vi "MST_softwareBin.vi"() -> ()   [LabVIEW 2012]
uses:
  <vilib>/addons/database/Auxilliary.llb/DB Tools Cursor Type.ctl
  <vilib>/Utility/NIReport.llb/NI_report.lvclass
  <vilib>/addons/database/Connection.llb/DB Tools Open Connec (Path).vi
  <vilib>/addons/database/Connection.llb/Conn Execute.vi
  <vilib>/addons/database/Recordset.llb/Rec Fetch Recordset Data (R).vi
  <vilib>/addons/database/Recordset.llb/Rec Destroy - Connection.vi
  <vilib>/Utility/NIReport.llb/Append Text Table to Report (wrap).vi
  <vilib>/addons/database/_DB Variant To Data/Database Variant To Data.xnode
  <vilib>/addons/database/NI_Database_API.lvlib
  <vilib>/Utility/NIReport.llb/Excel/NI_Excel.lvclass
panel:
  out "error out 2":errorcluster
  out "Row Headers":string[](array[string])
  in  "Report Template":path=path "O:/Monitor/Report/MSTsoftBin.xls"
  out "appended array":string[](array[string])
  out "data":string
  out "recordset data":variant[][](array[variant])
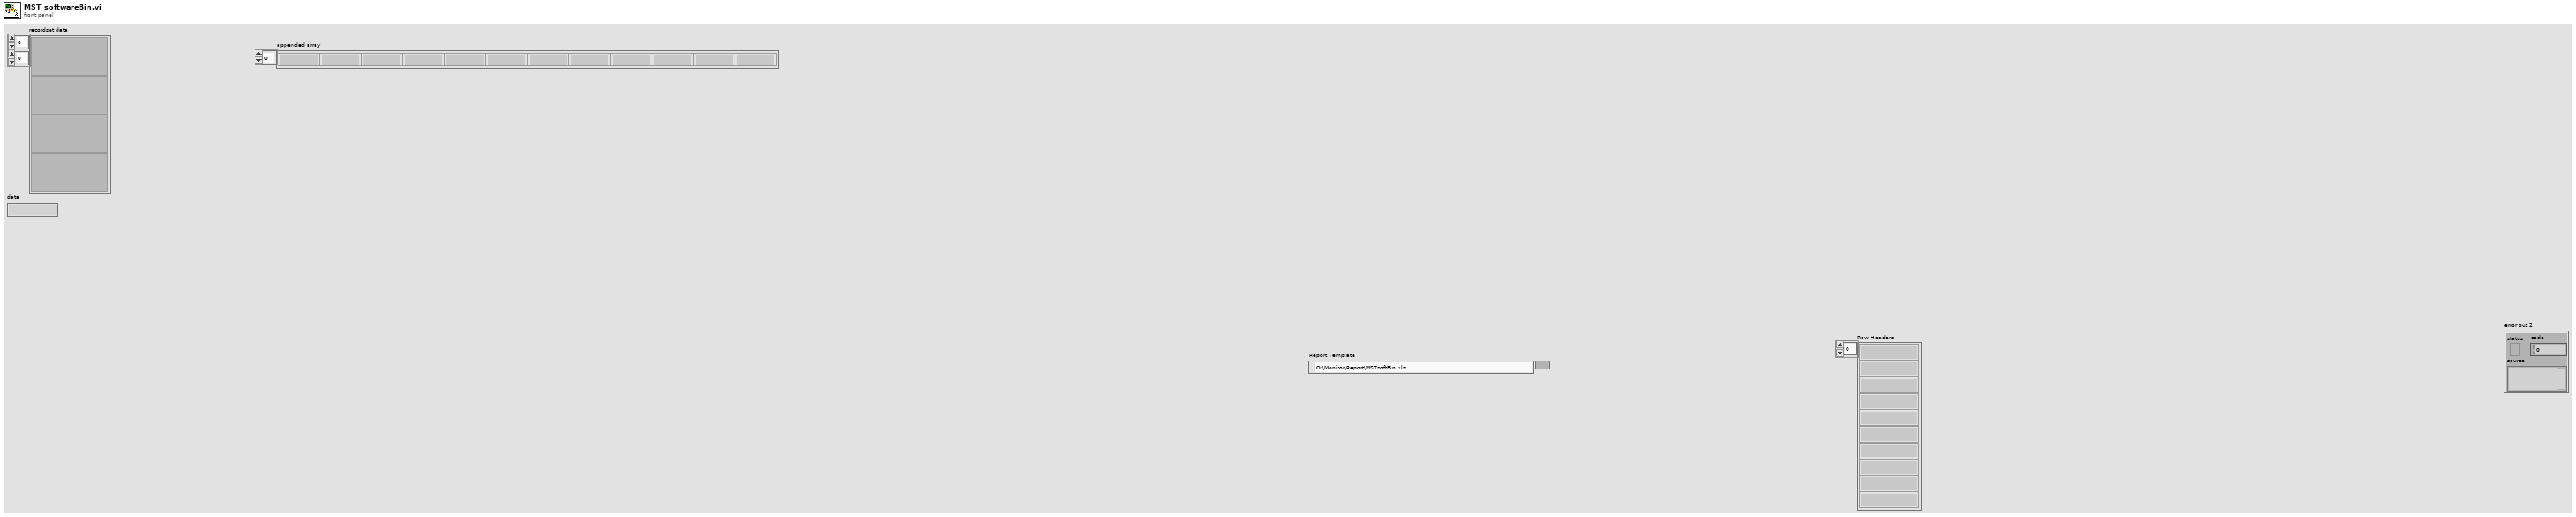
[diagram p1: front panel]
types:
  T1 = typedef "NI_Database_API.lvlib/DB Tools Cursor Type.ctl" = enum16{"forward-only", "keyset", "dynamic", "static"}
  T2 = enum16{"Standard Report", "HTML", "Word", "Excel"}
  T3 = typedef "NI_Database_API.lvlib/Conn ObjectReference.ctl" = refnum<k1>
  T4 = typedef "NI_Database_API.lvlib/Rec ObjectReference.ctl" = refnum<k1>
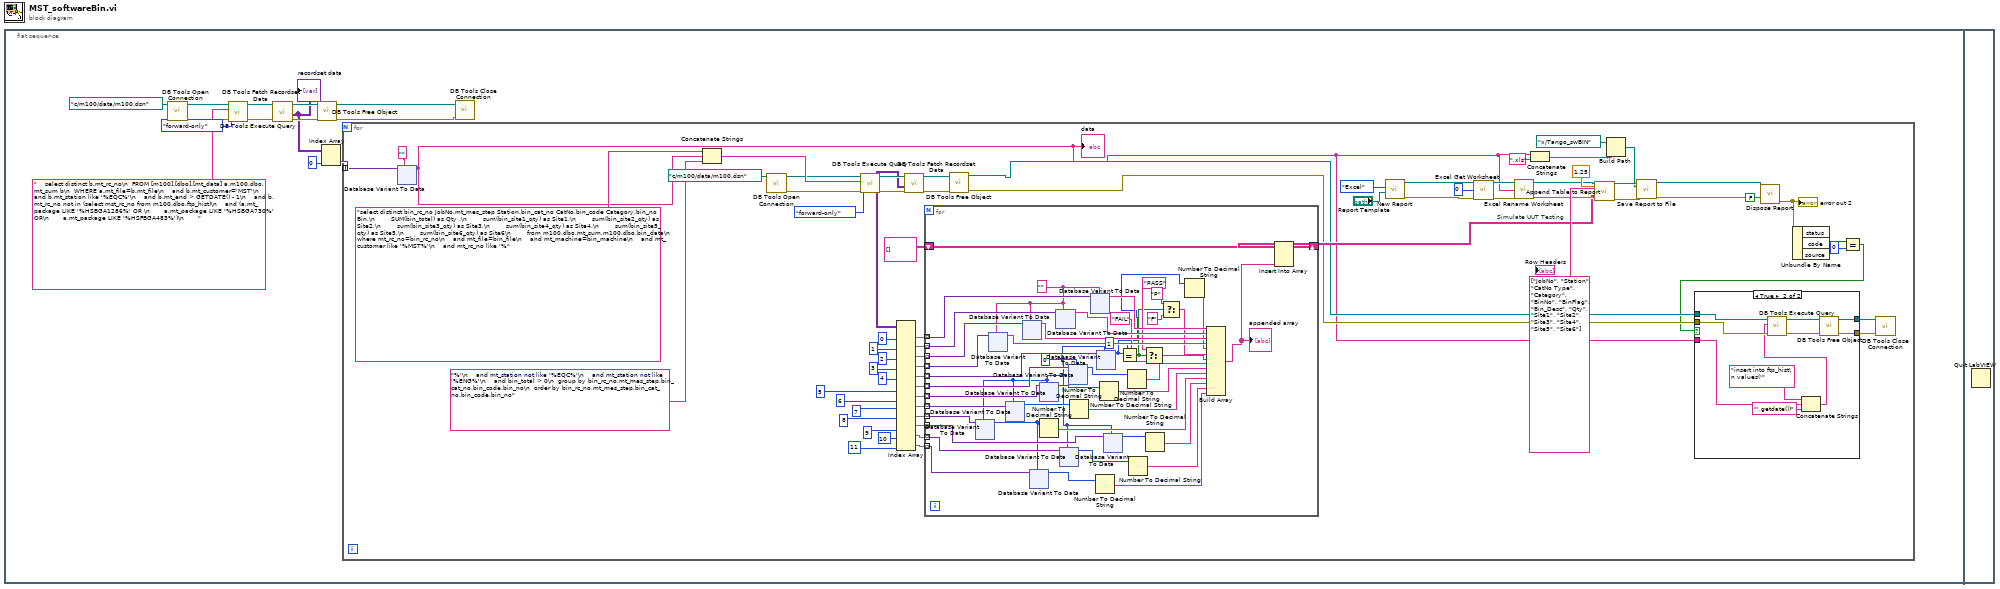
[diagram p0: block diagram]
diagram:
  n1 = flat-sequence {
    frame #0 {
      n2 = call-poly <vilib>:"DB Tools Open Connection.vi"("connection information"=path "c:/m100/data/m100.dsn") -> ("error out"=w11:errorcluster, "connection reference"=w14:T3)  [unwired: 7 in]
      n3 = call-poly <vilib>:"DB Tools Execute Query.vi"("error in (no error)"=w11, "cursor type"=DB_Tools_Cursor_Type."forward-only", "SQL query"="    select distinct b.mt_rc_no\n  FROM [m100].[dbo].[mt_data] a,m100.dbo.mt_sum b\n  WHERE a.mt_file=b.mt_file\n    and b.mt_customer='MST'\n    and b.mt_station like '%EQC%'\n    and b.mt_end > GETDATE() - 1\n    and b.mt_rc_no not in (select mst_rc_no from m100.dbo.ftp_hist)\n    and (a.mt_package LIKE '%HSBGA1286%' OR \n       a.mt_package LIKE '%HSBGA730%' OR\n       a.mt_package LIKE '%HSFBGA483%')\n       ", "connection reference"=w14) -> ("error out"=w10:errorcluster, "recordset reference"=w13:T4)  [unwired: 4 in]
      n4 = call-poly <vilib>:"DB Tools Fetch Recordset Data.vi"("error in (no error)"=w10, "recordset reference"=w13) -> ("error out"=w9:errorcluster, "recordset data"=w5:variant[][], "recordset reference out"=w12:T4)  [unwired: 3 in]
      "recordset data" <- w5
      n5 = call-poly <vilib>:"DB Tools Free Object.vi"("error in (no error)"=w9, "recordset reference"=w12) -> ("error out"=w1:errorcluster, "connection reference"=w2:T3)  [unwired: 8 in]
      n6 = Index Array(array=w5, index (col)=0 ("disabled index (col)")) -> (element=w3:variant[])  [unwired: 1 in]
      n7 = for {
        tunnel: w3 -> [w83] mode=indexing
        # "Simulate UUT Testing"
        n8 = xnode "Database Variant To Data"("database variant"=w83, "type"="") -> ("data"=w23:string)  [unwired: 1 in, 1 out]
        "data" <- w23
        n9 = Concatenate Strings("select distinct bin_rc_no JobNo,mt_mes_step Station,bin_cat_no CatNo,bin_code Category,bin_no Bin,\n        SUM(bin_total) as Qty ,\n        sum(bin_site1_qty) as Site1,\n        sum(bin_site2_qty) as Site2,\n        sum(bin_site3_qty) as Site3,\n        sum(bin_site4_qty) as Site4,\n        sum(bin_site5_qty) as Site5,\n        sum(bin_site6_qty) as Site6\n        from m100.dbo.mt_sum,m100.dbo.bin_data\n  where mt_rc_no=bin_rc_no\n    and mt_file=bin_file\n    and mt_machine=bin_machine\n    and mt_customer like '%MST%'\n    and mt_rc_no like '%" ("string"), w23, "%'\n    and mt_station not like '%EQC%'\n    and mt_station not like '%ENG%'\n    and bin_total > 0\n  group by bin_rc_no,mt_mes_step,bin_cat_no,bin_code,bin_no\n  order by bin_rc_no,mt_mes_step,bin_cat_no,bin_code,bin_no" ("string")) -> (w74:string)
        n10 = call-poly <vilib>:"DB Tools Open Connection.vi"("connection information"=path "c:/m100/data/m100.dsn") -> ("error out"=w18:errorcluster, "connection reference"=w19:T3)  [unwired: 7 in]
        n11 = call-poly <vilib>:"DB Tools Execute Query.vi"("error in (no error)"=w18, "cursor type"=DB_Tools_Cursor_Type."forward-only", "SQL query"=w74, "connection reference"=w19) -> ("error out"=w79:errorcluster, "recordset reference"=w81:T4)  [unwired: 4 in]
        n12 = call-poly <vilib>:"DB Tools Fetch Recordset Data.vi"("error in (no error)"=w79, "recordset reference"=w81) -> ("error out"=w78:errorcluster, "recordset data"=w73:variant[][], "recordset reference out"=w80:T4)  [unwired: 3 in]
        n13 = Index Array(array=w73, index (col) #1=0 ("disabled index (col)"), index (col) #2=1 ("index (col)"), index (col) #3=2 ("index (col)"), index (col) #4=3 ("index (col)"), index (col) #5=4 ("index (col)"), index (col) #6=5 ("index (col)"), index (col) #7=6 ("index (col)"), index (col) #8=7 ("index (col)"), index (col) #9=8 ("index (col)"), index (col) #10=9 ("index (col)"), index (col) #11=10 ("index (col)"), index (col) #12=11 ("index (col)")) -> (element #1=w62:variant[], element #2=w61:variant[], element #3=w60:variant[], element #4=w59:variant[], element #5=w58:variant[], element #6=w57:variant[], element #7=w56:variant[], element #8=w55:variant[], element #9=w54:variant[], element #10=w53:variant[], element #11=w50:variant[], element #12=w49:variant[])  [unwired: 12 in]
        n14 = for {
          tunnel: w62 -> [w140] mode=indexing
          tunnel: w61 -> [w139] mode=indexing
          tunnel: w60 -> [w138] mode=indexing
          tunnel: w59 -> [w137] mode=indexing
          tunnel: w58 -> [w136] mode=indexing
          tunnel: w57 -> [w135] mode=indexing
          tunnel: w56 -> [w134] mode=indexing
          tunnel: w55 -> [w133] mode=indexing
          tunnel: w54 -> [w132] mode=indexing
          tunnel: w53 -> [w131] mode=indexing
          tunnel: w50 -> [w121] mode=indexing
          tunnel: w49 -> [w120] mode=indexing
          shift-right: [w115] -> w36
          shift-left: string[][] [] ("array") -> [w114]
          w106 = 0
          w130 = ""
          n15 = xnode "Database Variant To Data"("database variant"=w132, "type"=w106) -> ("data"=w118:i32)  [unwired: 1 in, 1 out]
          n16 = xnode "Database Variant To Data"("database variant"=w137, "type"=w130) -> ("data"=w126:string)  [unwired: 1 in, 1 out]
          n17 = xnode "Database Variant To Data"("database variant"=w133, "type"=w106) -> ("data"=w123:i32)  [unwired: 1 in, 1 out]
          n18 = xnode "Database Variant To Data"("database variant"=w138, "type"=w130) -> ("data"=w127:string)  [unwired: 1 in, 1 out]
          n19 = xnode "Database Variant To Data"("database variant"=w120, "type"=w118) -> ("data"=w119:i32)  [unwired: 1 in, 1 out]
          n20 = Number To Decimal String(number=w118) -> (decimal integer string=w110:string)  [unwired: 1 in]
          n21 = xnode "Database Variant To Data"("database variant"=w134, "type"=w106) -> ("data"=w124:i32)  [unwired: 1 in, 1 out]
          n22 = xnode "Database Variant To Data"("database variant"=w139, "type"=w130) -> ("data"=w128:string)  [unwired: 1 in, 1 out]
          n23 = xnode "Database Variant To Data"("database variant"=w121, "type"=w106) -> ("data"=w117:i32)  [unwired: 1 in, 1 out]
          n24 = xnode "Database Variant To Data"("database variant"=w135, "type"=w106) -> ("data"=w125:i32)  [unwired: 1 in, 1 out]
          n25 = Number To Decimal String(number=w123) -> (decimal integer string=w109:string)  [unwired: 1 in]
          n26 = xnode "Database Variant To Data"("database variant"=w140, "type"=w130) -> ("data"=w129:string)  [unwired: 1 in, 1 out]
          n27 = Number To Decimal String(number=w119) -> (decimal integer string=w113:string)  [unwired: 1 in]
          n28 = xnode "Database Variant To Data"("database variant"=w136, "type"=w106) -> ("data"=w97:i32)  [unwired: 1 in, 1 out]
          n29 = Number To Decimal String(number=w124) -> (decimal integer string=w108:string)  [unwired: 1 in]
          n30 = xnode "Database Variant To Data"("database variant"=w131, "type"=w106) -> ("data"=w122:i32)  [unwired: 1 in, 1 out]
          n31 = Equal?(x=w97, y=1) -> (x = y?=w101:bool)
          n32 = Number To Decimal String(number=w125) -> (decimal integer string=w107:string)  [unwired: 1 in]
          n33 = Number To Decimal String(number=w117) -> (decimal integer string=w112:string)  [unwired: 1 in]
          n34 = Select(t="PASS", s=w101, f="FAIL") -> (s? t:f=w102:string)
          n35 = Number To Decimal String(number=w122) -> (decimal integer string=w111:string)  [unwired: 1 in]
          n36 = Select(t="P", s=w101, f="F") -> (s? t:f=w98:string)
          n37 = Number To Decimal String(number=w97) -> (decimal integer string=w96:string)  [unwired: 1 in]
          n38 = Build Array(w129, w128, w127, w126, w96, w98, w102, w107, w108, w109, w110, w111, w112, w113) -> (w116:string[])
          "appended array" <- w116
          n39 = Insert Into Array(array=w114, new element=w116) -> (w115:string[][])  [unwired: 2 in]
        }
        n40 = call-poly <vilib>:"DB Tools Free Object.vi"("error in (no error)"=w78, "recordset reference"=w80) -> ("error out"=w24:errorcluster, "connection reference"=w25:T3)  [unwired: 8 in]
        n41 = call <vilib>:"New Report.vi"("report type"=T2."Excel" ("Report Type"), "template (empty)"="Report Template") -> ("report out"=w43:refnum<class "NI_report.lvclass">, "error out"=w42:errorcluster)  [unwired: 12 in]
        n42 = call <vilib>:"Excel Get Worksheet.vi"("report in"=w43, "worksheet index (0)"=0, "error in (no error)"=w42) -> ("report out"=w40:refnum<class "NI_report.lvclass">, "error out"=w38:errorcluster)  [unwired: 11 in]
        n43 = call <vilib>:"Excel Rename Worksheet.vi"("report in"=w40, "worksheet name (\"\")"=w23, "error in (no error)"=w38) -> ("report out"=w39:refnum<class "NI_report.lvclass">, "error out"=w37:errorcluster)  [unwired: 11 in]
        n44 = Concatenate Strings(w23, ".xls" ("string")) -> (w29:string)
        n45 = call-poly <vilib>:"Append Table to Report.vi"("report in"=w39, "column width (1)"=1.25, "column headers"=string[] ["JobNo", "Station", "CatNo Type", "Category", "BinNo", "BinFlag", "Bin_Desc", "Qty", "Site1", "Site2", "Site3", "Site4", "Site5", "Site6"] ("row headers"), "text data"=w36, "error in (no error)"=w37) -> ("report out"=w32:refnum<class "NI_report.lvclass">, "error out"=w31:errorcluster)  [unwired: 7 in, 2 out]
        n46 = Build Path(base path=path "x:/Tango_swBIN", name or relative path=w29) -> (appended path=w27:path)
        n47 = call-dynamic "Save Report to File.vi"("report in"=w32, "report file path"=w27, "error in (no error)"=w31) -> ("report out"=w34:refnum<class "NI_report.lvclass">, "error out"=w33:errorcluster)  [unwired: 11 in]
        n48 = call-dynamic "Dispose Report.vi"("report in"=w34, "save changes? (F)"=FALSE, "error in (no error)"=w33) -> ("error out"=w26:errorcluster)  [unwired: 12 in]
        "error out 2" <- w26
        n49 = Unbundle By Name(w26) -> ("code"=w22:i32)  [unwired: 2 out]
        n50 = Equal?(x=w22, y=0) -> (x = y?=w20:bool)
        n51 = case shown="True" w20 {
          tunnel: w25 -> [w85 w95]
          tunnel: w24 -> [w84 w94]
          tunnel: w23 -> [_ w92]
          tunnel: [w85 w87] -> w16
          tunnel: [w84 w86] -> w15
          frame False {
          }
          frame True {
            n52 = Concatenate Strings("insert into ftp_hist\n values('" ("string"), w92, "',getdate())" ("string")) -> (w90:string)
            n53 = call-poly <vilib>:"DB Tools Execute Query.vi"("error in (no error)"=w94, "SQL query"=w90, "connection reference"=w95) -> ("error out"=w88:errorcluster, "recordset reference"=w89:T4)  [unwired: 5 in]
            n54 = call-poly <vilib>:"DB Tools Free Object.vi"("error in (no error)"=w88, "recordset reference"=w89) -> ("error out"=w86:errorcluster, "connection reference"=w87:T3)  [unwired: 8 in]
          }
        }
        n55 = call <vilib>:"DB Tools Close Connection.vi"("error in (no error)"=w15, "connection reference"=w16) -> ()  [unwired: 5 in, 1 out]
      }
      n56 = call <vilib>:"DB Tools Close Connection.vi"("error in (no error)"=w1, "connection reference"=w2) -> ()  [unwired: 5 in, 1 out]
    }
    frame #1 {
      n57 = Quit LabVIEW() -> ()  [unwired: 1 in]
    }
  }
